vi "Realsense Cam Wrapper Connect.vi"(8 "error in (no error)":errorcluster, 11 "Realsense Cam Wrapper in":refnum<class "Realsense Cam Wrapper.lvclass">) -> (0 "error out":errorcluster, 1 "Found?":bool, 2 "init error":string, 3 "Realsense Cam Wrapper out":refnum<class "Realsense Cam Wrapper.lvclass">)   [LabVIEW 2018, in "Realsense Cam Wrapper.lvclass"]
uses:
  Realsense Cam Wrapper.lvclass
  Temp/realsense_labview_sdk/RealSense SDK2.11.0 for LabVIEW/libRealSense3.lvlib
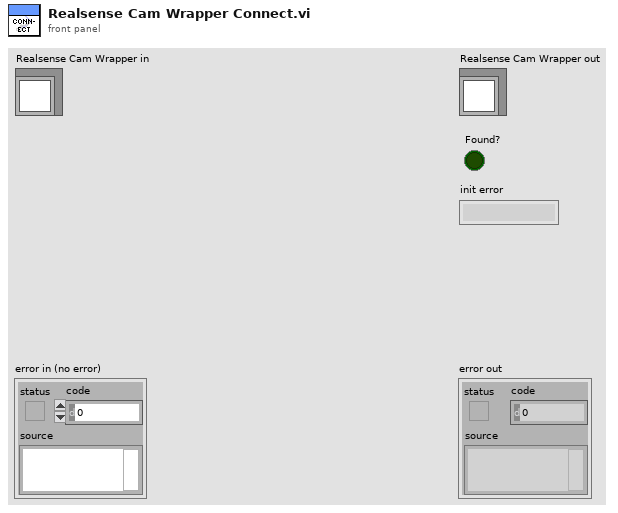
[diagram p1: front panel]
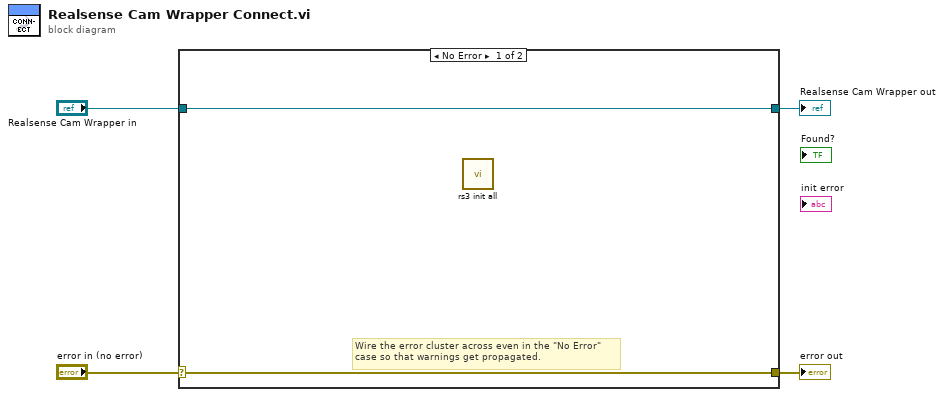
[diagram p0: block diagram]
diagram:
  n1 = case shown="No Error" "error in (no error)" {
    selector: "error in (no error)" -> [w5 w8]
    tunnel: [w5 w8] -> w3
    tunnel: [w6 w7] -> w1
    tunnel: "Realsense Cam Wrapper in" -> [w6 w7]
    frame No Error {
      # "Wire the error cluster across even in the \"No Error\"\ncase so that warnings get propagated."
      n2 = call "rs3 init all.vi"() -> ()  [unwired: 5 in, 7 out]
    }
    frame Error {
    }
  }
  "error out" <- w3
  "Realsense Cam Wrapper out" <- w1
